vi "Trim Whitespace Lookup Table.vi"() -> ()   [LabVIEW 2023, in "openg_string.lvlib"]
uses:
  openg_string.lvlib
panel:
  out "ASCII Whitespace Lookup Table":bool[](array[boolean])
  # "Generate ASCII Whitespace Lookup Table\n\nSee Block Diagram from details"
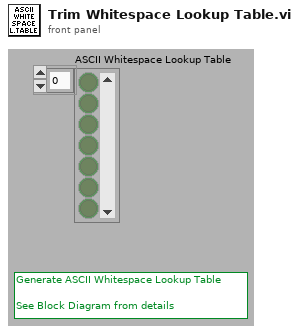
[diagram p1: front panel]
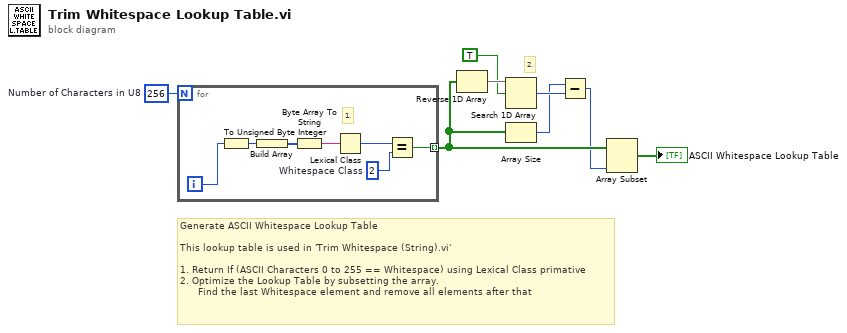
[diagram p0: block diagram]
diagram:
  w8 = 256  # Number of Characters in U8
  # "2."
  # "Generate ASCII Whitespace Lookup Table\n\nThis lookup table is used in 'Trim Whitespace (String).vi'\n\n1. Return If (ASCII Characters 0 to 255 == Whitespace) using Lexical Class primative\n2. Optimize the Lookup Table by subsetting the array.\n      Find the last Whitespace element and remove all elements after that"
  n1 = for {
    N: w8 -> [_]
    tunnel: [w10] -> w3 mode=indexing
    i -> [w9]
    w11 = i16 2  # Whitespace Class
    # "1."
    n2 = To Unsigned Byte Integer(number=w9) -> (unsigned 8bit integer=w14:u8)
    n3 = Build Array(w14) -> (w15:u8[])
    n4 = Byte Array To String(unsigned byte array=w15) -> (string=w13:string)
    n5 = Lexical Class(1:w13) -> (0:w12:i16)
    n6 = Equal?(x=w12, y=w11) -> (x = y?=w10:bool)
  }
  n7 = Reverse 1D Array(array=w3) -> (reversed array=w6:bool[])
  n8 = Search 1D Array(1D array=w6, element=TRUE) -> (index of element=w4:i32)  [unwired: 1 in]
  n9 = Array Size(array=w3) -> (size(s)=w2:i32)
  n10 = Subtract(x=w2, y=w4) -> (x-y=w1:i32)
  n11 = Array Subset(array=w3, length=w1) -> (→"ASCII Whitespace Lookup Table":bool[])  [unwired: 1 in]
